vi "AlliGator_Graphs Metadata Types.vi"(11 "Graph Label":string) -> (1 "Found?":bool, 3 "Plot Metadata Type":variant)   [LabVIEW 2021, in "AlliGator GUI.lvlib"]
uses:
  Lifetime & Other Parameters Graph Metadata.ctl
  GUI/AlliGator GUI.lvlib
  Lifetime & Other Parameters/AlliGator Lifetime & Other Parameters.lvlib
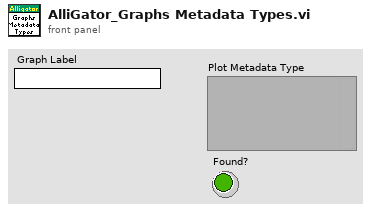
[diagram p1: front panel]
types:
  T1 = typedef "AlliGator Lifetime & Other Parameters.lvlib/Lifetime & Other Parameters Graph Metadata.ctl" = cluster{"Intensity Array":sgl[]}[]
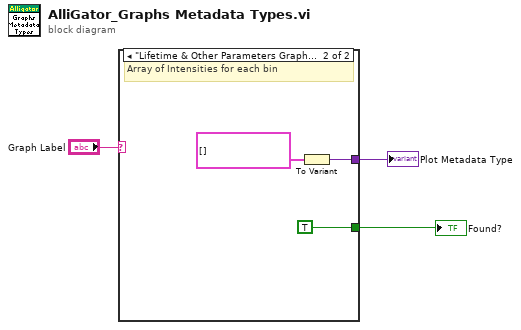
[diagram p0: block diagram]
diagram:
  n1 = case shown="\"Lifetime & Other Parameters Graph\"" "Graph Label" {
    tunnel: [_ w5] -> w2
    tunnel: [_ TRUE ("Found?")] -> w1
    frame "", Default {
    }
    frame "Lifetime & Other Parameters Graph" {
      # "Array of Intensities for each bin"
      n2 = To Variant(anything=T1 []) -> (Variant=w5:variant)
    }
  }
  "Plot Metadata Type" <- w2
  "Found?" <- w1
